vi "SetFunctionArbs.vi"(8 "error in (no error)":errorcluster, 10 "Variant":variant, 11 "PmuTestFunctions in":refnum<class "PmuTestFunctions.lvclass">) -> (0 "error out":errorcluster, 3 "PmuTestFunctions out":refnum<class "PmuTestFunctions.lvclass">)   [LabVIEW 2018, in "Functions.lvlib" / "PmuTestFunctions.lvclass"]
uses:
  PmuTestFunctions.lvclass
  PmuTestFunctions.lvclass/PmuTestFunctions.ctl
  Accessors/Write SettlingTime.vi
  Accessors/Write T0.vi
  ArbitraryFunction/ArbitraryFunction.lvclass
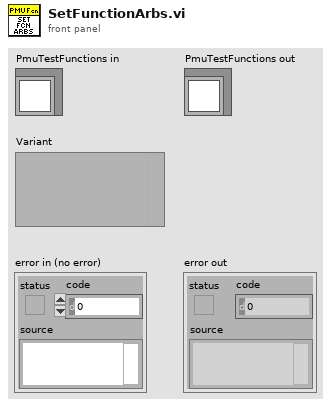
[diagram p1: front panel]
types:
  T1 = cluster{"Arbs":cluster{"Handle":string, "Size":i32, "Gain":dbl, "Offset":dbl}[], "SampleRate":dbl, "SettlingTime":dbl, "T0":dbl}
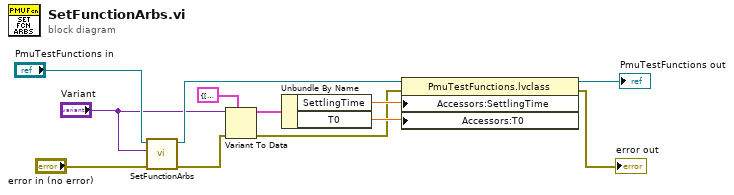
[diagram p0: block diagram]
diagram:
  n1 = call-parent "SetFunctionArbs.vi"("error in (no error)"="error in (no error)", "Variant"="Variant", "ArbitraryFunction in"="PmuTestFunctions in") -> ("error out"=w7:errorcluster, "ArbitraryFunction out"=w12:refnum<class "PmuTestFunctions.lvclass">)  [unwired: 7 in]
  n2 = Variant To Data(error in=w7, type=T1 {"Arbs"=[], "SampleRate"=0.0, "SettlingTime"=0.0, "T0"=0.0} ("FunctionConfig"), Variant="Variant") -> (data=w6:T1, error out=w2:errorcluster)
  n3 = Unbundle By Name(w6) -> ("SettlingTime"=w4:dbl, "T0"=w3:dbl)
  n4 = property class="PmuTestFunctions.lvclass"(reference=w12, error in=w2, "Accessors:SettlingTime"=w4, "Accessors:T0"=w3) -> (reference out=→"PmuTestFunctions out":refnum<class "PmuTestFunctions.lvclass">, error out=→"error out":errorcluster)
